vi "Image Processing with Vision Assistant (FPGA)-useFIFO.vi"() -> ()   [LabVIEW 2016]
uses:
  <vilib>/visionFPGA/Controls/IMAQ FPGA Image Size.ctl
  <vilib>/rvi/Emulation/niFpgaSctlEmulationGetInTimedLoop.vi
  <vilib>/rvi/Emulation/niFpgaProcessEmulError.vi
  <vilib>/rvi/Emulation/niFpgaGetClockAttributes.vi
  <vilib>/rvi/Emulation/niFpgaEmulationReportErrorSimple.vi
  <vilib>/rvi/eio/common/nirviEmuTemplateMethod_errors.vi
  <vilib>/rvi/interface/RandomDataEmulation/niFpgaRandomDataHandleErrors.vi
  <vilib>/rvi/DataTransferAndStorage/Container/Common/niFpgaContainerGetUniqueNameForEmu.vi
  <vilib>/rvi/DataTransferAndStorage/Container/Common/niFpgaContainerSetEmuInfo.vi
  <vilib>/rvi/eio/common/nirviEmuReportErrorAndStop.vi
  <vilib>/rvi/DataTransferAndStorage/Container/Common/niFpgaContainerExecOnDevCompGetState.vi
  <vilib>/rvi/Emulation/niFpgaEmulationIsFPGAContextNoSignature.vi
  <vilib>/rvi/errors/niFpgaSetErrorForExecOnDevCompSimple.vi
  <vilib>/rvi/FIFO/Fifo_Resource/nirvififoEmulationSetSize.vi
  <vilib>/rvi/FIFO/Fifo_Resource/nirviFifoEmulationQueueMgr.vi
  <instcachedir>/0/nirviFifoEmulationQueueMgr_E5CAEC123FF24DC58D834DCA3CDAA9B5.lvgen/nirviFifoEmulationQueueMgr_E5CAEC123FF24DC58D834DCA3CDAA9B5_002.vi
  <vilib>/rvi/FIFO/Fifo_Resource/nirvififoEmulationDetermineInputValidOut.vi
  <vilib>/rvi/FIFO/Fifo_Resource/nirvififoEmulationCreateLock.vi
  <vilib>/rvi/FIFO/Fifo_Resource/nirvififoEmulationObtainLock.vi
  <vilib>/rvi/FIFO/Fifo_Resource/nirvififoEmulationReleaseLock.vi
  <vilib>/rvi/occurrence/nirviWaitOnOccurrenceBase.vi
  <vilib>/rvi/errors/nirviReportUnexpectedCaseInternalError.vi
  <vilib>/rvi/errors/nirviReportUnexpectedCaseInternalError (U32).vi
  <vilib>/Utility/error.llb/Clear Errors.vi
  <vilib>/rvi/Emulation/niFpgaCriticalErrorInLSC.vi
  <vilib>/eio/EIONode/EIONode.xnode
  <vilib>/rvi/DataTransferAndStorage/Container/XNode/niFpgaContainer.xnode
  <vilib>/rvi/interface/RandomDataEmulation/nirviRandomDataFpgaReadWriteTemplate.vi
  <vilib>/rvi/LocalResourceManager/LocalResourceManager.xnode
  <vilib>/rvi/FIFO/Fifo_Resource/niFpgaFifoEmulationRefIn.vi
panel:
  out "deHeight":u16=240
  out "deWidth":u16=320
  out "Count":u32
  out "OutputType":u8
  out "CanSendImage":bool=TRUE
  out "Mode LED Status":bool=TRUE
  out "Radio LED Status":bool=TRUE
  out "outputExtreme2":bool=TRUE
  out "outputExtreme1":bool=TRUE
  out "outputDOG2":bool=TRUE
  out "outputDOG1":bool=TRUE
  out "Ready For Output":bool=TRUE
  out "StartOfImage":bool=TRUE
  in  "Image Size":T1={"Width"=640, "Height"=480}
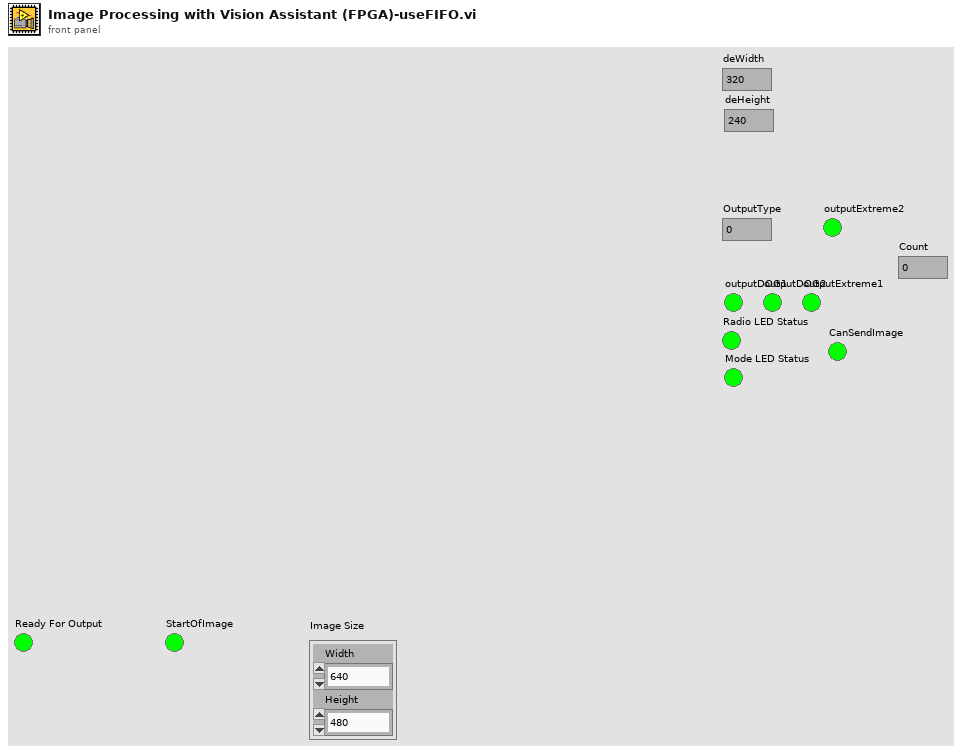
[diagram p1: front panel]
types:
  T1 = typedef "IMAQ FPGA Image Size.ctl" = cluster{"Width":u32, "Height":u32}
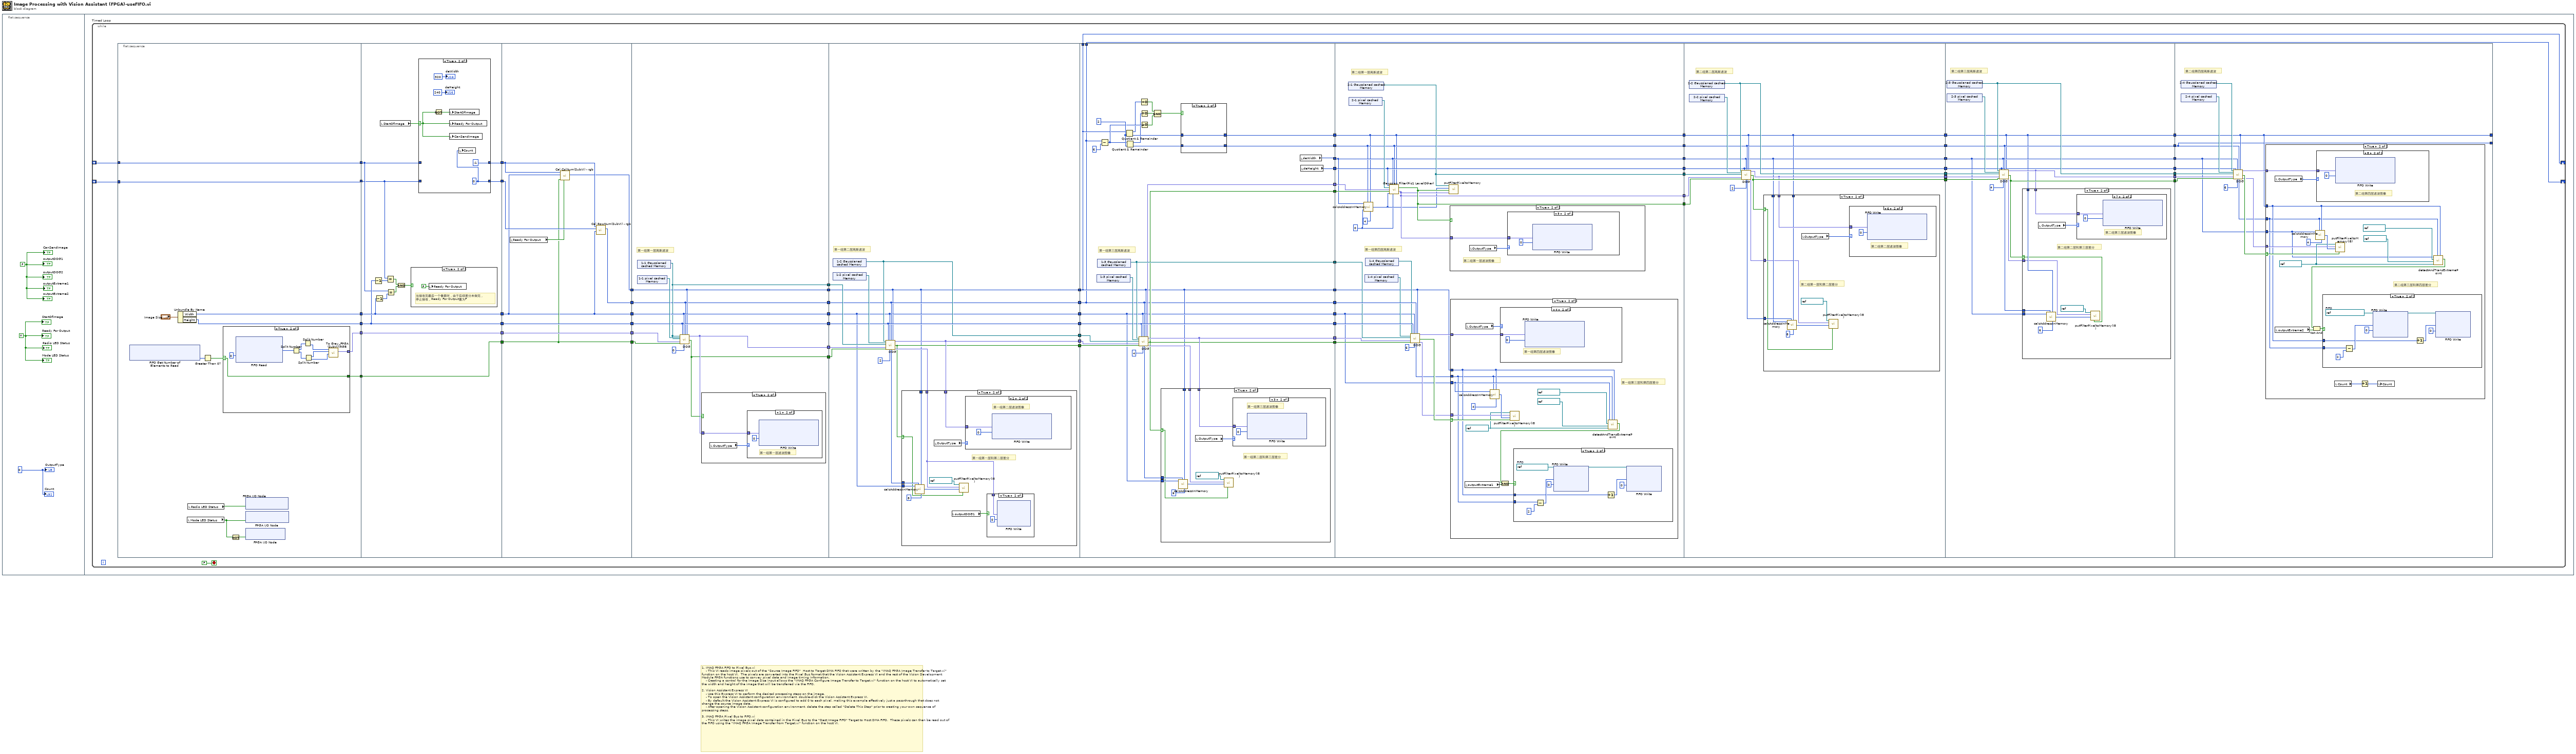
[diagram p0: block diagram]
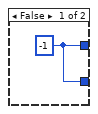
[diagram p10: hidden frame]
diagram:
  # "1. IMAQ FPGA FIFO to Pixel Bus.vi\n    - This VI reads image pixels out of the \"Source Image FIFO\"  Host to Target DMA FIFO that were written by the \"IMAQ FPGA Image Transfer to Target.vi\" function on the host VI.  The pixels are converted into the Pixel Bus format that the Vision Assistant Express VI and the rest of the Vision Development Module FPGA functions use to convey pixel data and image timing information.\n    - Creating a control for the Image Size input allows the \"IMAQ FPGA Configure Image Transfer to Target.vi\" function on the host VI to automatically set the width and height of the image that will be transferred via the FIFO.\n\n2. Vision Assistant Express VI\n    - Use this Express VI to perform the desired processing steps on the image.\n    - To open the Vision Assistant configuration environment, double-click the Vision Assistant Express VI.\n    - By default the Vision Assistant Express VI is configured to add 0 to each pixel, making this example effectively just a pass-through that does not change the source image data.\n    - After opening the Vision Assistant configuration environment, delete the step called \"Delete This Step\" prior to creating your own sequence of processing steps.\n\n3. IMAQ FPGA Pixel Bus to FIFO.vi\n    - This VI writes the image pixel data contained in the Pixel Bus to the \"Dest Image FIFO\" Target to Host DMA FIFO.  These pixels can then be read out of the FIFO using the \"IMAQ FPGA Image Transfer from Target.vi\" function on the host VI."
  n1 = flat-sequence {
    frame #0 {
      w1 = FALSE
      w2 = i16 0
      w3 = TRUE ("Ready For Output")
      "StartOfImage" <- w3
      "Ready For Output" <- w3
      "outputDOG1" <- w1
      "outputDOG2" <- w1
      "outputExtreme1" <- w1
      "outputExtreme2" <- w1
      "Radio LED Status" <- w3
      "Mode LED Status" <- w3
      "CanSendImage" <- w1
      "OutputType" <- w2
      "Count" <- w2
    }
    frame #1 {
      n2 = while "Timed Loop" {
        shift-right: [w10] -> _
        shift-left: _ -> [w14]
        shift-right: [w11] -> _
        shift-left: _ -> [w16]
        stop <- FALSE stop-if-true
        n3 = flat-sequence {
          tunnel: [w85] -> w21
          tunnel: [w84] -> w20
          tunnel: [w78] -> w19
          tunnel: [w77] -> w18
          tunnel: [w76] -> w17
          tunnel: w16 -> [w76]
          tunnel: [w75] -> w15
          tunnel: w14 -> [w75]
          tunnel: [w105] -> w26
          tunnel: [w103] -> w25
          tunnel: [w102] -> w24
          tunnel: [w104] -> w23
          tunnel: w21 -> [w103]
          tunnel: w20 -> [w102]
          tunnel: w19 -> [w105]
          tunnel: w18 -> [w104]
          tunnel: w17 -> [w100]
          tunnel: w15 -> [w99]
          tunnel: [w98] -> w13
          tunnel: [w97] -> w12
          tunnel: [w121] -> w4
          tunnel: [w128] -> w8
          tunnel: [w122] -> w6
          tunnel: [w127] -> w7
          tunnel: [w123] -> w9
          tunnel: w26 -> [w128]
          tunnel: w25 -> [w122]
          tunnel: w24 -> [w127]
          tunnel: w23 -> [w123]
          tunnel: w13 -> [w125]
          tunnel: w12 -> [w126]
          tunnel: [w120] -> w5
          tunnel: w9 -> [w129]
          tunnel: w8 -> [w139]
          tunnel: w7 -> [w135]
          tunnel: w6 -> [w136]
          tunnel: w5 -> [w131]
          tunnel: w4 -> [w130]
          tunnel: [w131] -> w74
          tunnel: [w130] -> w73
          tunnel: [w136] -> w72
          tunnel: [w135] -> w71
          tunnel: [w138] -> w70
          tunnel: [w132] -> w69
          tunnel: [w133] -> w66
          tunnel: w74 -> [w144]
          tunnel: w73 -> [w150]
          tunnel: w72 -> [w146]
          tunnel: w71 -> [w152]
          tunnel: w70 -> [w154]
          tunnel: w69 -> [w153]
          tunnel: [w147] -> w68
          tunnel: [w149] -> w67
          tunnel: w66 -> [w155]
          tunnel: [w144] -> w65
          tunnel: [w150] -> w64
          tunnel: [w146] -> w63
          tunnel: [w152] -> w62
          tunnel: [w151] -> w54
          tunnel: w68 -> [w201]
          tunnel: w67 -> [w200]
          tunnel: w65 -> [w176]
          tunnel: w64 -> [w175]
          tunnel: w63 -> [w177]
          tunnel: w62 -> [w194]
          tunnel: [w181] -> w61
          tunnel: [w179] -> w60
          tunnel: [w176] -> w59
          tunnel: [w175] -> w58
          tunnel: [w177] -> w57
          tunnel: [w194] -> w56
          tunnel: [w198] -> w55
          tunnel: w54 -> [w197]
          tunnel: [w174] -> w53
          tunnel: [w173] -> w52
          tunnel: [w187] -> w51
          tunnel: [w188] -> w50
          tunnel: [w181] -> w49
          tunnel: [w179] -> w48
          tunnel: [w176] -> w11
          tunnel: [w175] -> w10
          tunnel: w61 -> [w243]
          tunnel: w60 -> [w242]
          tunnel: w59 -> [w220]
          tunnel: w58 -> [w241]
          tunnel: w57 -> [w222]
          tunnel: w56 -> [w240]
          tunnel: w55 -> [w237]
          tunnel: w53 -> [w229]
          tunnel: w52 -> [w230]
          tunnel: w51 -> [w228]
          tunnel: w50 -> [w227]
          tunnel: w49 -> [w232]
          tunnel: w48 -> [w233]
          tunnel: [w235] -> w47
          tunnel: [w225] -> w46
          tunnel: [w226] -> w45
          tunnel: [w230] -> w44
          tunnel: [w229] -> w43
          tunnel: [w228] -> w42
          tunnel: [w227] -> w41
          tunnel: w47 -> [w285]
          tunnel: w46 -> [w284]
          tunnel: w45 -> [w283]
          tunnel: w44 -> [w281]
          tunnel: w43 -> [w274]
          tunnel: w42 -> [w280]
          tunnel: w41 -> [w276]
          tunnel: [w282] -> w40
          tunnel: [w276] -> w39
          tunnel: [w280] -> w38
          tunnel: [w274] -> w37
          tunnel: [w281] -> w36
          tunnel: [w277] -> w35
          tunnel: [w279] -> w34
          tunnel: w40 -> [w311]
          tunnel: w39 -> [w300]
          tunnel: w38 -> [w307]
          tunnel: w37 -> [w302]
          tunnel: w36 -> [w306]
          tunnel: w35 -> [w310]
          tunnel: w34 -> [w309]
          tunnel: [w304] -> w33
          tunnel: [w305] -> w32
          tunnel: [w308] -> w31
          tunnel: [w300] -> w30
          tunnel: [w307] -> w29
          tunnel: [w302] -> w28
          tunnel: [w306] -> w27
          tunnel: w33 -> [w336]
          tunnel: w32 -> [w335]
          tunnel: w31 -> [w334]
          tunnel: w30 -> [w327]
          tunnel: w29 -> [w326]
          tunnel: w28 -> [w329]
          tunnel: w27 -> [w333]
          tunnel: [w327] -> _
          tunnel: [w326] -> _
          frame #0 {
            n4 = xnode ("FIFO Get Number of Elements to Read")() -> ("Number of Elements to Read"=w80:u32)  [unwired: 1 in, 1 out]
            n5 = Unbundle By Name("Image Size") -> ("Width"=w85:u32, "Height"=w84:u32)
            n6 = local read "Mode LED Status"() -> (w83:bool)
            n7 = local read "Radio LED Status"() -> (w81:bool)
            n8 = Greater Than 0?(x=w80) -> (x > 0?=w79:bool)
            n9 = case shown="True" w79 {
              selector: w79 -> [w87 w88]
              tunnel: [_ w89] -> w78
              tunnel: [w87 w88] -> w77
              frame False {
              }
              frame True {
                n10 = xnode ("FIFO Read")("Timeout"=0) -> ("Element"=w96:u32)  [unwired: 1 in, 2 out]
                n11 = Split Number(x=w96) -> (hi(x)=w94:u16, lo(x)=w95:u16)
                n12 = Split Number(x=w94) -> (lo(x)=w93:u8)  [unwired: 1 out]
                n13 = Split Number(x=w95) -> (hi(x)=w92:u8, lo(x)=w91:u8)
                n14 = call "To Gray_FPGA (SubVI)-RGB.vi"("B"=w91, "G"=w92, "R"=w93) -> ("Data Out"=w89:fxp<+,8,8>)  [unwired: 8 in]
              }
            }
            n15 = Not(x=w83) -> (.not. x?=w82:bool)
            n16 = xnode "FPGA I/O Node"("Radio LED Green"=w81) -> ()  [unwired: 1 in, 1 out]
            n17 = xnode "FPGA I/O Node"("Mode LED Green"=w83) -> ()  [unwired: 1 in, 1 out]
            n18 = xnode "FPGA I/O Node"("Mode LED Red"=w82) -> ()  [unwired: 1 in, 1 out]
          }
          frame #1 {
            n19 = Decrement(x=w102) -> (x-1=w108:u32)
            n20 = Decrement(x=w103) -> (x-1=w107:u32)
            n21 = local read "StartOfImage"() -> (w101:bool)
            n22 = Equal?(x=w99, y=w108) -> (x = y?=w110:bool)
            n23 = Equal?(x=w100, y=w107) -> (x = y?=w109:bool)
            n24 = And(x=w110, y=w109) -> (x .and. y?=w106:bool)
            n25 = case shown="True" w106 {
              frame False {
              }
              frame True {
                # "当接收完最后一个像素时，由于后续差分未做完，\n停止接收，Ready For Output置为F"
                n26 = local write "Ready For Output"(FALSE ("Ready For Output")) -> ()
              }
            }
            n27 = case shown="True" w101 {
              selector: w101 -> [_ w116]
              tunnel: w100 -> [w112 _]
              tunnel: w99 -> [w111 _]
              tunnel: [w112 i16 -1] -> w98
              tunnel: [w111 w115] -> w97
              frame False {
              }
              frame True {
                w115 = i16 0
                n28 = Not(x=w116) -> (.not. x?=w117:bool)
                n29 = local write "StartOfImage"(w117) -> ()
                n30 = local write "Ready For Output"(w116) -> ()
                n31 = local write "CanSendImage"(w116) -> ()
                n32 = local write "Count"(w115) -> ()
                "deWidth" <- i16 320
                "deHeight" <- i16 240
              }
            }
          }
          frame #2 {
            n33 = local read "Ready For Output"() -> (w124:bool)
            n34 = call "Cal ColNum(SubVI) - rgb.vi"("Ready For Input"=w124, "DV"=w123, "Width"=w122, "preCol"=w125) -> ("curCol"=w120:u16)  [unwired: 7 in]
            n35 = call "Cal RowNum(SubVI) - rgb.vi"("Width"=w122, "preRow"=w126, "preCol"=w125) -> ("curRow"=w121:u16)  [unwired: 8 in]
          }
          frame #3 {
            # "第一组第一层高斯滤波"
            n36 = xnode "1-1 Gaussianed cached Memory"() -> ("Memory Out"=w133:refnum<k21>)
            n37 = xnode "1-1 pixel cached Memory"() -> ("Memory Out"=w137:refnum<k21>)
            n38 = call "DOG.vi"("Gaussianed cached Memory"=w133, "pixel cached Memory"=w137, "preGaussianed cached Memory"=w133, "Data in"=w139, "DV in"=w129, "Height"=w135, "Width"=w136, "DelayRowCount"=i16 0, "Rows"=w130, "Cols"=w131) -> ("GaussianFilterData out"=w138:fxp<+,12,12>, "DV out"=w132:bool)  [unwired: 6 in, 2 out]
            n39 = case shown="True" w132 {
              tunnel: w138 -> [_ w141]
              frame False {
              }
              frame True {
                n40 = local read "OutputType"() -> (w140:u8)
                n41 = case shown="1" w140 {
                  tunnel: w141 -> [_ w142]
                  frame 0, Default {
                  }
                  frame 1 {
                    # "第一组第一层滤波图像"
                    n42 = xnode ("FIFO Write")("Element"=w142, "Timeout"=0) -> ()  [unwired: 1 in, 2 out]
                  }
                }
              }
            }
          }
          frame #4 {
            # "第一组第二层高斯滤波"
            n43 = xnode "1-2 Gaussianed cached Memory"() -> ("Memory Out"=w151:refnum<k21>)
            n44 = xnode "1-2 pixel cached Memory"() -> ("Memory Out"=w156:refnum<k21>)
            n45 = call "DOG.vi"("Gaussianed cached Memory"=w151, "pixel cached Memory"=w156, "preGaussianed cached Memory"=w155, "Data in"=w154, "DV in"=w153, "Height"=w152, "Width"=w146, "DelayRowCount"=i16 2, "Rows"=w150, "Cols"=w144) -> ("out Row"=w145:u16, "GaussianFilterData out"=w149:fxp<+,12,12>, "DV out"=w147:bool, "DOG Out"=w148:fxp<+/-,13,13>)  [unwired: 6 in]
            n46 = case shown="True" w147 {
              selector: w147 -> [_ w161]
              tunnel: w149 -> [_ w168]
              tunnel: w148 -> [_ w159]
              tunnel: w146 -> [_ w167]
              tunnel: w145 -> [_ w166]
              tunnel: w144 -> [_ w165]
              frame False {
              }
              frame True {
                # "第一组第一层和第二层差分"
                n47 = call "calcAddressInMemory.vi"("Width"=w167, "Rows"=w166, "Cols"=w165, "divider"=u8 8) -> ("addressInMemory"=w163:u16)  [unwired: 5 in]
                n48 = local read "OutputType"() -> (w160:u8)
                n49 = local read "outputDOG1"() -> (w158:bool)
                n50 = call "putFilterPixeltoMemory(I8).vi"("DV in"=w161, "addressInMemory"=w163, "Data In"=w159, "Memory in"=refnum<k21> "DOG1-1") -> ()  [unwired: 8 in]
                n51 = case shown="2" w160 {
                  tunnel: w168 -> [_ w171]
                  frame 0, Default {
                  }
                  frame 2 {
                    # "第一组第二层滤波图像"
                    n52 = xnode ("FIFO Write")("Element"=w171, "Timeout"=0) -> ()  [unwired: 1 in, 2 out]
                  }
                }
                n53 = case shown="True" w158 {
                  tunnel: w159 -> [_ w170]
                  frame False {
                  }
                  frame True {
                    n54 = xnode ("FIFO Write")("Element"=w170, "Timeout"=0) -> ()  [unwired: 1 in, 2 out]
                  }
                }
              }
            }
          }
          frame #5 {
            w193 = u32 2 ("y")
            # "第一组第三层高斯滤波"
            n55 = xnode "1-3 pixel cached Memory"() -> ("Memory Out"=w199:refnum<k21>)
            n56 = xnode "1-3 Gaussianed cached Memory"() -> ("Memory Out"=w198:refnum<k21>)
            n57 = Subtract(x=w175, y=i16 6) -> (x-y=w184:u16)
            n58 = Quotient & Remainder(x=w176, y=w193) -> (x-y*floor(x/y)=w183:u32, floor(x/y)=w185:u32)
            n59 = Quotient & Remainder(x=w184, y=w193) -> (x-y*floor(x/y)=w182:u32, floor(x/y)=w186:u32)
            n60 = call "DOG.vi"("Gaussianed cached Memory"=w198, "pixel cached Memory"=w199, "preGaussianed cached Memory"=w197, "Data in"=w200, "DV in"=w201, "Height"=w194, "Width"=w177, "DelayRowCount"=i16 4, "Rows"=w175, "Cols"=w176) -> ("out Row"=w178:u16, "GaussianFilterData out"=w181:fxp<+,12,12>, "DV out"=w179:bool, "DOG Out"=w180:fxp<+/-,13,13>)  [unwired: 6 in]
            n61 = Equal To 0?(x=w183) -> (x = 0?=w192:bool)
            n62 = Equal To 0?(x=w182) -> (x = 0?=w191:bool)
            n63 = Greater Or Equal To 0?(x=w184) -> (x >= 0?=w190:bool)
            n64 = Compound Arithmetic op=AND(w192, w191, w190) -> (w189:bool)
            n65 = case shown="True" w179 {
              selector: w179 -> [_ w206]
              tunnel: w181 -> [_ w214]
              tunnel: w180 -> [_ w207]
              tunnel: w178 -> [_ w210]
              tunnel: w177 -> [_ w209]
              tunnel: w176 -> [_ w208]
              frame False {
              }
              frame True {
                # "第一组第二层和第三层差分"
                n66 = call "calcAddressInMemory.vi"("Width"=w209, "Rows"=w210, "Cols"=w208, "divider"=u8 6) -> ("addressInMemory"=w212:u16)  [unwired: 5 in]
                n67 = local read "OutputType"() -> (w205:u8)
                n68 = call "putFilterPixeltoMemory(I8).vi"("DV in"=w206, "addressInMemory"=w212, "Data In"=w207, "Memory in"=refnum<k21> "DOG1-2") -> ()  [unwired: 8 in]
                n69 = case shown="3" w205 {
                  tunnel: w214 -> [_ w215]
                  frame 0, Default {
                  }
                  frame 3 {
                    # "第一组第三层滤波图像"
                    n70 = xnode ("FIFO Write")("Element"=w215, "Timeout"=0) -> ()  [unwired: 1 in, 2 out]
                  }
                }
              }
            }
            n71 = case shown="True" w189 {
              tunnel: [w202 w204] -> w188
              tunnel: w185 -> [_ w204]
              tunnel: [w202 w203] -> w187
              tunnel: w186 -> [_ w203]
              frame False {
                w202 = i16 -1 ("t")
              }
              frame True {
              }
            }
            n72 = local read "deWidth"() -> (w174:u16)
            n73 = local read "deHeight"() -> (w173:u16)
          }
          frame #6 {
            w218 = u8 0 ("delayRowCount")
            # "第二组第一层高斯滤波"
            # "第一组第四层高斯滤波"
            n74 = xnode "2-1 Gaussianed cached Memory"() -> ("Memory Out"=w235:refnum<k21>)
            n75 = xnode "2-1 pixel cached Memory"() -> ("Memory Out"=w231:refnum<k21>)
            n76 = call "calcAddressInMemory.vi"("Width"=w229, "Rows"=w228, "delayRowCount"=w218, "Cols"=w227, "divider"=u8 4) -> ("addressInMemory"=w219:u16)  [unwired: 4 in]
            n77 = xnode "1-4 pixel cached Memory"() -> ("Memory Out"=w238:refnum<k21>)
            n78 = xnode "1-4 Gaussianed cached Memory"() -> ("Memory Out"=w239:refnum<k21>)
            n79 = call "Gaussian Filter(Pic1 LevelOther).vi"("Height"=w230, "Width"=w229, "Rows"=w228, "Cols"=w227, "Memory in"=w231, "Data in"=w232, "DV in"=w233, "Address In"=w219, "DelayRowCount"=w218) -> ("DV out"=w226:bool, "Data Out"=w225:fxp<+,8,8>)  [unwired: 4 in, 1 out]
            n80 = call "DOG.vi"("Gaussianed cached Memory"=w239, "pixel cached Memory"=w238, "preGaussianed cached Memory"=w237, "Data in"=w243, "DV in"=w242, "Height"=w240, "Width"=w222, "DelayRowCount"=i16 6, "Rows"=w241, "Cols"=w220) -> ("out Row"=w221:u16, "GaussianFilterData out"=w234:fxp<+,12,12>, "DV out"=w224:bool, "DOG Out"=w223:fxp<+/-,13,13>)  [unwired: 6 in]
            n81 = call "putFilterPixeltoMemory.vi"("Data In"=w225, "DV in"=w226, "addressInMemory"=w219, "Memory in"=w235) -> ()
            n82 = case shown="True" w226 {
              tunnel: w225 -> [_ w245]
              frame False {
              }
              frame True {
                # "第二组第一层滤波图像"
                n83 = local read "OutputType"() -> (w244:u8)
                n84 = case shown="5" w244 {
                  tunnel: w245 -> [_ w246]
                  frame 0, Default {
                  }
                  frame 5 {
                    n85 = xnode ("FIFO Write")("Element"=w246, "Timeout"=0) -> ()  [unwired: 1 in, 2 out]
                  }
                }
              }
            }
            n86 = case shown="True" w224 {
              selector: w224 -> [_ w258]
              tunnel: w234 -> [_ w262]
              tunnel: w223 -> [_ w259]
              tunnel: w222 -> [_ w257]
              tunnel: w221 -> [_ w251]
              tunnel: w220 -> [_ w252]
              frame False {
              }
              frame True {
                w254 = refnum<k21> "DOG1-3" ("Memory in")
                # "第一组第三层和第四层差分"
                n87 = local read "outputExtreme1"() -> (w249:bool)
                n88 = local read "OutputType"() -> (w253:u8)
                n89 = call "calcAddressInMemory.vi"("Width"=w257, "Rows"=w251, "Cols"=w252, "divider"=u8 4) -> ("addressInMemory"=w260:u16)  [unwired: 5 in]
                n90 = case shown="4" w253 {
                  tunnel: w262 -> [_ w273]
                  frame 0, Default {
                  }
                  frame 4 {
                    # "第一组第四层滤波图像"
                    n91 = xnode ("FIFO Write")("Element"=w273, "Timeout"=0) -> ()  [unwired: 1 in, 2 out]
                  }
                }
                n92 = call "putFilterPixeltoMemory(I8).vi"("DV in"=w258, "addressInMemory"=w260, "Data In"=w259, "Memory in"=w254) -> ()  [unwired: 8 in]
                n93 = call "detectAndTransExtremePoint.vi"("Col"=w252, "Row"=w251, "Level3 Memory"=w254, "Level2 Memory"=refnum<k21> "DOG1-2" ("Memory In"), "Level1 Memory"=refnum<k21> "DOG1-1" ("Memory In"), "Width"=w257) -> ("isExtreme?"=w248:bool)  [unwired: 5 in]
                n94 = And(x=w248, y=w249) -> (x .and. y?=w250:bool)
                n95 = case shown="True" w250 {
                  tunnel: w251 -> [_ w270]
                  tunnel: w252 -> [_ w264]
                  frame False {
                  }
                  frame True {
                    w263 = refnum<k21> "extreme FIFO"  # FIFO
                    n96 = Subtract(x=w270, y=u16 2) -> (x-y=w268:u16)
                    n97 = xnode ("FIFO Write")("Element"=w268, "Timeout"=0, "FIFO In"=w263) -> ("FIFO Out"=w266:refnum<k21>)  [unwired: 1 out]
                    n98 = Increment(x=w264) -> (x+1=w265:u16)
                    n99 = xnode ("FIFO Write")("Element"=w265, "Timeout"=0, "FIFO In"=w266) -> ()  [unwired: 2 out]
                  }
                }
              }
            }
          }
          frame #7 {
            # "第二组第二层高斯滤波"
            n100 = xnode "2-2 Gaussianed cached Memory"() -> ("Memory Out"=w282:refnum<k21>)
            n101 = xnode "2-2 pixel cached Memory"() -> ("Memory Out"=w286:refnum<k21>)
            n102 = call "DOG.vi"("Gaussianed cached Memory"=w282, "pixel cached Memory"=w286, "preGaussianed cached Memory"=w285, "Data in"=w284, "DV in"=w283, "Height"=w281, "Width"=w274, "DelayRowCount"=i16 2, "Rows"=w280, "Cols"=w276) -> ("out Row"=w275:u16, "GaussianFilterData out"=w277:fxp<+,12,12>, "DV out"=w279:bool, "DOG Out"=w278:fxp<+/-,13,13>)  [unwired: 6 in]
            n103 = case shown="True" w279 {
              selector: w279 -> [_ w289]
              tunnel: w278 -> [_ w290]
              tunnel: w277 -> [_ w297]
              tunnel: w276 -> [_ w293]
              tunnel: w275 -> [_ w292]
              tunnel: w274 -> [_ w291]
              frame False {
              }
              frame True {
                # "第二组第一层和第二层差分"
                n104 = call "calcAddressInMemory.vi"("Width"=w291, "Rows"=w292, "Cols"=w293, "divider"=u8 8) -> ("addressInMemory"=w295:u16)  [unwired: 5 in]
                n105 = local read "OutputType"() -> (w288:u8)
                n106 = call "putFilterPixeltoMemory(I8).vi"("DV in"=w289, "addressInMemory"=w295, "Data In"=w290, "Memory in"=refnum<k21> "DOG2-1") -> ()  [unwired: 8 in]
                n107 = case shown="6" w288 {
                  tunnel: w297 -> [_ w298]
                  frame 0, Default {
                  }
                  frame 6 {
                    # "第二组第二层滤波图像"
                    n108 = xnode ("FIFO Write")("Element"=w298, "Timeout"=0) -> ()  [unwired: 1 in, 2 out]
                  }
                }
              }
            }
          }
          frame #8 {
            # "第二组第三层高斯滤波"
            n109 = xnode "2-3 Gaussianed cached Memory"() -> ("Memory Out"=w308:refnum<k21>)
            n110 = xnode "2-3 pixel cached Memory"() -> ("Memory Out"=w312:refnum<k21>)
            n111 = call "DOG.vi"("Gaussianed cached Memory"=w308, "pixel cached Memory"=w312, "preGaussianed cached Memory"=w311, "Data in"=w310, "DV in"=w309, "Height"=w306, "Width"=w302, "DelayRowCount"=i16 4, "Rows"=w307, "Cols"=w300) -> ("out Row"=w301:u16, "GaussianFilterData out"=w304:fxp<+,12,12>, "DV out"=w305:bool, "DOG Out"=w303:fxp<+/-,13,13>)  [unwired: 6 in]
            n112 = case shown="True" w305 {
              selector: w305 -> [_ w315]
              tunnel: w304 -> [_ w323]
              tunnel: w303 -> [_ w316]
              tunnel: w302 -> [_ w319]
              tunnel: w301 -> [_ w318]
              tunnel: w300 -> [_ w317]
              frame False {
              }
              frame True {
                # "第二组第二层和第三层差分"
                n113 = local read "OutputType"() -> (w314:u8)
                n114 = call "calcAddressInMemory.vi"("Width"=w319, "Rows"=w318, "Cols"=w317, "divider"=u8 6) -> ("addressInMemory"=w321:u16)  [unwired: 5 in]
                n115 = case shown="7" w314 {
                  tunnel: w323 -> [_ w325]
                  frame 0, Default {
                  }
                  frame 7 {
                    # "第二组第三层滤波图像"
                    n116 = xnode ("FIFO Write")("Element"=w325, "Timeout"=0) -> ()  [unwired: 1 in, 2 out]
                  }
                }
                n117 = call "putFilterPixeltoMemory(I8).vi"("DV in"=w315, "addressInMemory"=w321, "Data In"=w316, "Memory in"=refnum<k21> "DOG2-2") -> ()  [unwired: 8 in]
              }
            }
          }
          frame #9 {
            # "第二组第四层高斯滤波"
            n118 = xnode "2-4 Gaussianed cached Memory"() -> ("Memory Out"=w337:refnum<k21>)
            n119 = xnode "2-4 pixel cached Memory"() -> ("Memory Out"=w338:refnum<k21>)
            n120 = call "DOG.vi"("Gaussianed cached Memory"=w337, "pixel cached Memory"=w338, "preGaussianed cached Memory"=w334, "Data in"=w336, "DV in"=w335, "Height"=w333, "Width"=w329, "DelayRowCount"=i16 6, "Rows"=w326, "Cols"=w327) -> ("out Row"=w328:u16, "GaussianFilterData out"=w331:fxp<+,12,12>, "DV out"=w332:bool, "DOG Out"=w330:fxp<+/-,13,13>)  [unwired: 6 in]
            n121 = case shown="True" w332 {
              selector: w332 -> [_ w350]
              tunnel: w331 -> [_ w356]
              tunnel: w330 -> [_ w349]
              tunnel: w329 -> [_ w348]
              tunnel: w328 -> [_ w346]
              tunnel: w327 -> [_ w347]
              frame False {
              }
              frame True {
                w351 = refnum<k21> "DOG2-3" ("Memory in")
                # "第二组第三层和第四层差分"
                n122 = local read "OutputType"() -> (w342:u8)
                n123 = local read "outputExtreme2"() -> (w343:bool)
                n124 = call "calcAddressInMemory.vi"("Width"=w348, "Rows"=w346, "Cols"=w347, "divider"=u8 4) -> ("addressInMemory"=w354:u16)  [unwired: 5 in]
                n125 = case shown="8" w342 {
                  tunnel: w356 -> [_ w358]
                  frame 0, Default {
                  }
                  frame 8 {
                    # "第二组第四层滤波图像"
                    n126 = xnode ("FIFO Write")("Element"=w358, "Timeout"=0) -> ()  [unwired: 1 in, 2 out]
                  }
                }
                n127 = local read "Count"() -> (w341:u32)
                n128 = call "putFilterPixeltoMemory(I8).vi"("DV in"=w350, "addressInMemory"=w354, "Data In"=w349, "Memory in"=w351) -> ()  [unwired: 8 in]
                n129 = Increment(x=w341) -> (x+1=w340:u32)
                n130 = local write "Count"(w340) -> ()
                n131 = call "detectAndTransExtremePoint.vi"("Col"=w347, "Row"=w346, "Level3 Memory"=w351, "Level2 Memory"=refnum<k21> "DOG2-2" ("Memory In"), "Level1 Memory"=refnum<k21> "DOG2-1" ("Memory In"), "Width"=w348) -> ("isExtreme?"=w344:bool)  [unwired: 5 in]
                n132 = Not And(1:w343, 2:w344) -> (0:w345:bool)
                n133 = case shown="True" w345 {
                  tunnel: w346 -> [_ w366]
                  tunnel: w347 -> [_ w360]
                  frame False {
                  }
                  frame True {
                    w359 = refnum<k21> "extreme FIFO dec"  # FIFO
                    n134 = Subtract(x=w366, y=u16 2) -> (x-y=w364:u16)
                    n135 = xnode ("FIFO Write")("Element"=w364, "Timeout"=0, "FIFO In"=w359) -> ("FIFO Out"=w362:refnum<k21>)  [unwired: 1 out]
                    n136 = Increment(x=w360) -> (x+1=w361:u32)
                    n137 = xnode ("FIFO Write")("Element"=w361, "Timeout"=0, "FIFO In"=w362) -> ()  [unwired: 2 out]
                  }
                }
              }
            }
          }
        }
      }
    }
  }
